vi "Update and Error.vi"(7 "Time":timestamp, 8 "Data":map{string, dbl}(c390), 9 "error IO":errorcluster, 10 "Key":string) -> (0 "error out":errorcluster)   [LabVIEW 2024, in "IOLink.lvlib"]
uses:
  IOLink.lvlib
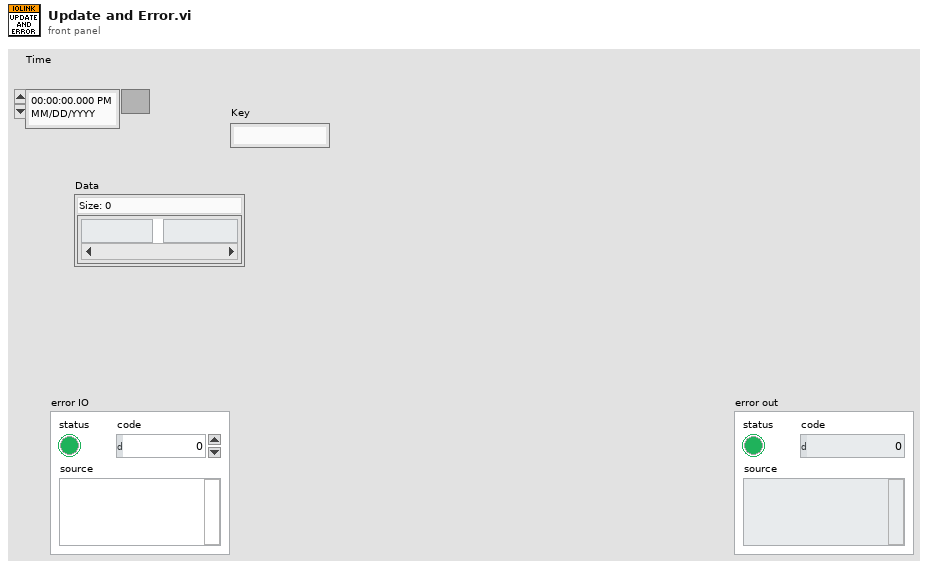
[diagram p1: front panel]
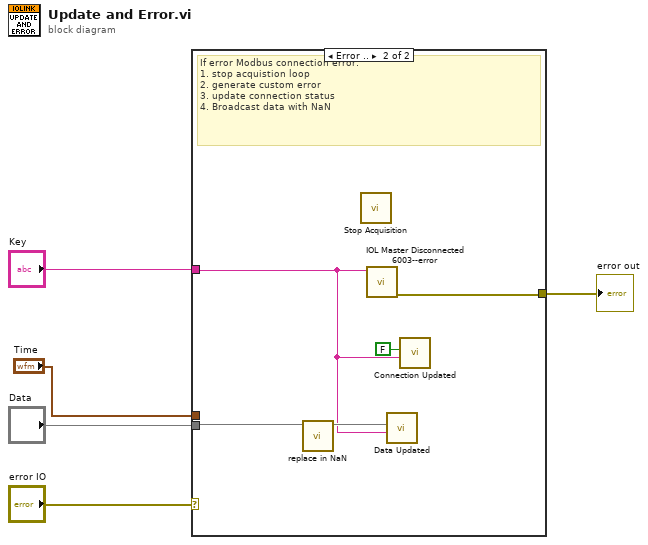
[diagram p0: block diagram]
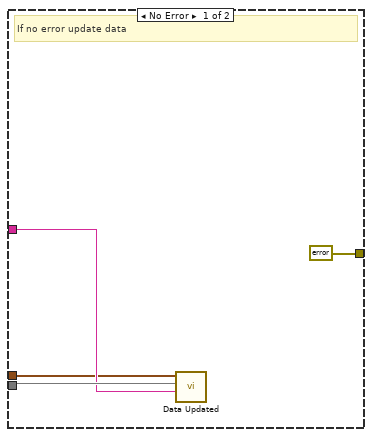
[diagram p2: hidden frame]
diagram:
  n1 = case shown="Error .." "error IO" {
    tunnel: "Data" -> [w8 w13]
    tunnel: "Key" -> [w7 w10]
    tunnel: [errorcluster {"status"=FALSE, "code"=0, "source"=""} ("error out") w14] -> w2
    tunnel: "Time" -> [w6 _]
    frame No Error {
      # "If no error update data"
      n2 = call "Data Updated.vi"("Key"=w7, "Data"=w8, "Time"=w6) -> ()  [unwired: 8 in, 1 out]
    }
    frame Error {
      # "If error Modbus connection error:\n1. stop acquistion loop\n2. generate custom error\n3. update connection status\n4. Broadcast data with NaN"
      n3 = call "replace in NaN.vi"("Data In"=w13) -> ("Data Out"=w12:map{string, dbl})  [unwired: 10 in]
      n4 = call "Stop Acquisition.vi"() -> ()  [unwired: 11 in, 1 out]
      n5 = call "IOL Master Disconnected 6003--error.vi"("Master Key"=w10) -> ("error out"=w14:errorcluster)  [unwired: 10 in]
      n6 = call "Data Updated.vi"("Key"=w10, "Data"=w12) -> ()  [unwired: 9 in, 1 out]
      n7 = call "Connection Updated.vi"("Key"=w10, "Connection State"=FALSE) -> ()  [unwired: 9 in, 1 out]
    }
  }
  "error out" <- w2
